vi "RT Main-采集AI数据.vi"() -> ()   [LabVIEW 2019]
uses:
  <vilib>/userdefined/High Color/nirio_resource_hc.ctl
  <vilib>/FPGAPlugInAG/ELVIS III/niLvFpga_Open_ELVIS III.vi
  <vilib>/rvi/interface/common/dynamic/niFpgaDynamicAddResources.vi
  <vilib>/Utility/error.llb/Error Cluster From Error Code.vi
  <vilib>/rvi/errors/niLvFpgaAdjustHostInterfaceError.vi
  <vilib>/rvi/interface/common/niFpgaWaitOnOcc.vi
  <vilib>/FPGAPlugInAG/Dynamic/niLvFpga_Run_Dynamic.vi
  <vilib>/measure/maspectr.llb/FFT Spectrum (Real-Im) for 1 Chan.vi
  <vilib>/FPGAPlugInAG/Dynamic/niLvFpga_Close_Dynamic.vi
  <vilib>/rvi/interface/nirviOpenFPGA/nirviOpenFPGA.xnode
  FPGA-Main.vi
  <vilib>/rvi/interface/nirviReadWriteControl/nirviReadWriteControl.xnode
  <vilib>/rvi/interface/nirviMethod/nirviMethod.xnode
  <vilib>/rvi/interface/nirviCloseFPGA/nirviCloseFPGA.xnode
  NiFpgaLv.dll
  <vilib>/rvi/interface/Simulation/niFpgaSimulationCallBeginRW.vi
  <vilib>/FPGAPlugInAG/Dynamic/niLvFpga_ConfigureFifo_Dynamic.vi
  <vilib>/rvi/errors/niLvFpgaMergeErrorWithErrorCode.vi
  <vilib>/FPGAPlugInAG/Dynamic/niLvFpga_ReadFifo_Dynamic.vi
  <vilib>/measure/NI_MAPro.lvlib
panel:
  in  "停止":bool
  out "波形图表 2":waveform(dbl)(graph)
  out "波形图表":waveform(dbl)(graph)
  in  "资源名称":T1="RIO0"
  in  "Count(uSec)":u32=10
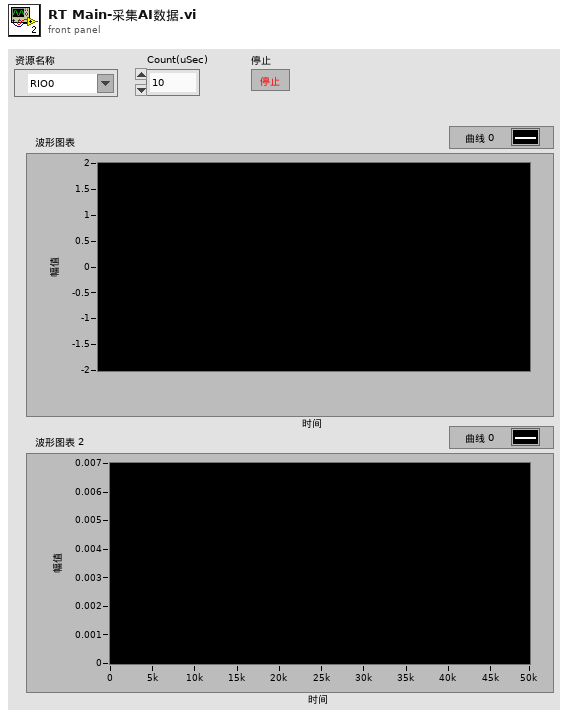
[diagram p1: front panel]
types:
  T1 = typedef "nirio_resource_hc.ctl" = tag
  T2 = cluster{"f0":dbl, "df":dbl, "imaginary part":dbl[]}
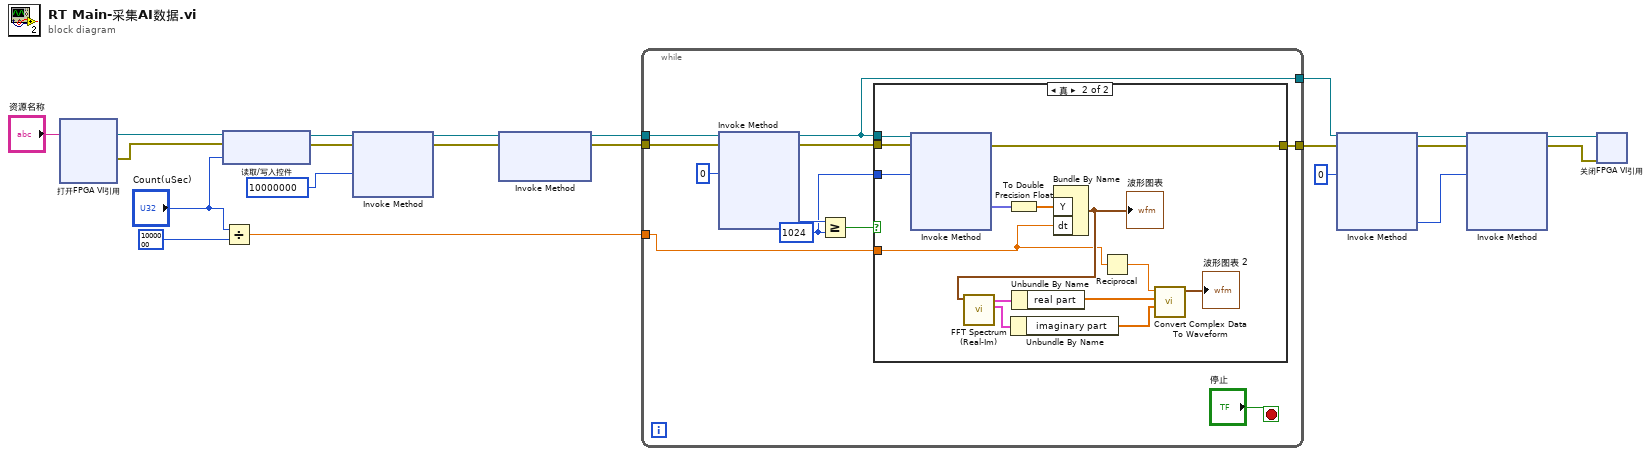
[diagram p0: block diagram]
diagram:
  n1 = xnode "打开FPGA VI引用"("资源名称"="资源名称") -> ("FPGA VI引用输出"=w20:refnum<k20>, "错误输出"=w21:errorcluster)  [unwired: 1 in]
  n2 = xnode "读取/写入控件"("FPGA VI引用输入"=w20, "错误输入"=w21, "Count(uSec)"="Count(uSec)") -> ("FPGA VI引用输出"=w19:refnum<k20>, "错误输出"=w18:errorcluster)
  n3 = Divide(x="Count(uSec)", y=u32 1000000) -> (x/y=w9:dbl)
  n4 = xnode "Invoke Method"("FPGA VI引用输入"=w19, "错误输入"=w18, "请求的深度"=u32 10000000) -> ("FPGA VI引用输出"=w14:refnum<k20>, "错误输出"=w15:errorcluster)  [unwired: 1 out]
  n5 = xnode "Invoke Method"("FPGA VI引用输入"=w14, "错误输入"=w15) -> ("FPGA VI引用输出"=w13:refnum<k20>, "错误输出"=w12:errorcluster)  [unwired: 1 in]
  n6 = while {
    tunnel: w13 -> [w31]
    tunnel: w12 -> [w32]
    tunnel: w9 -> [w25]
    tunnel: [w24] -> w8
    tunnel: [w23] -> w7
    stop <- "停止" stop-if-true
    w26 = u32 1024 ("y")
    n7 = xnode "Invoke Method"("FPGA VI引用输入"=w31, "错误输入"=w32, "元素数量"=u32 0) -> ("FPGA VI引用输出"=w23:refnum<k20>, "错误输出"=w27:errorcluster, "剩余元素"=w29:u32)  [unwired: 1 in, 1 out]
    n8 = Greater Or Equal?(x=w29, y=w26) -> (x >= y?=w28:bool)
    n9 = case shown="真" w28 {
      tunnel: w23 -> [_ w46]
      tunnel: w27 -> [w33 w47]
      tunnel: w26 -> [_ w45]
      tunnel: w25 -> [_ w36]
      tunnel: [w33 w44] -> w24
      frame False {
      }
      frame True {
        n10 = xnode "Invoke Method"("FPGA VI引用输入"=w46, "错误输入"=w47, "元素数量"=w45) -> ("错误输出"=w44:errorcluster, "数据"=w43:fxp<+/-,24,5>[])  [unwired: 1 in, 2 out]
        n11 = To Double Precision Float(number=w43) -> (double precision float=w42:dbl[])
        n12 = Bundle By Name("Y"=w42, "dt"=w36) -> (w41:waveform(dbl))  [unwired: 1 in]
        "波形图表" <- w41
        n13 = call-poly <vilib>:"FFT Spectrum (Real-Im).vi"("time signal"=w41) -> ("imaginary part"=w39:T2, "real part"=w40:cluster{"f0":dbl, "df":dbl, "real part":dbl[]})  [unwired: 6 in, 3 out]
        n14 = Unbundle By Name(w39) -> ("imaginary part"=w37:dbl[])
        n15 = Unbundle By Name(w40) -> ("real part"=w38:dbl[])
        n16 = Reciprocal(x=w36) -> (1/x=w35:dbl)
        n17 = call "Convert Complex Data To Waveform.vi"("Real Data"=w37, "Imaginary Data"=w38, "Sample Rate (S/s)"=w35) -> ("Waveform"=→"波形图表 2":waveform(dbl))  [unwired: 7 in, 1 out]
      }
    }
  }
  n18 = xnode "Invoke Method"("FPGA VI引用输入"=w7, "错误输入"=w8, "元素数量"=u32 0) -> ("FPGA VI引用输出"=w6:refnum<k20>, "错误输出"=w5:errorcluster, "剩余元素"=w3:u32)  [unwired: 1 in, 1 out]
  n19 = xnode "Invoke Method"("FPGA VI引用输入"=w6, "错误输入"=w5, "元素数量"=w3) -> ("FPGA VI引用输出"=w1:refnum<k20>, "错误输出"=w2:errorcluster)  [unwired: 1 in, 2 out]
  n20 = xnode "关闭FPGA VI引用"("FPGA VI引用输入"=w1, "错误输入"=w2) -> ()  [unwired: 1 out]
